vi "set_number_of_channels.vi"(8 "error in (no error)":errorcluster, 10 "number of channels":i32, 11 "GenericImageProcessor.lvclass in":refnum<class "GenericImageProcessor.lvclass">) -> (0 "error out":errorcluster, 3 "GenericImageProcessor.lvclass out":refnum<class "GenericImageProcessor.lvclass">)   [LabVIEW 2010, in "GenericImageProcessor.lvclass"]
uses:
  GenericImageProcessor.lvclass
  GenericImageProcessor.lvclass/GenericImageProcessor.ctl
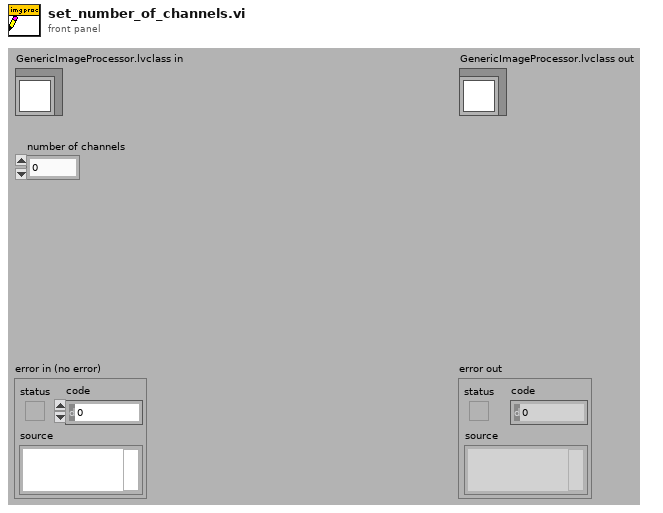
[diagram p1: front panel]
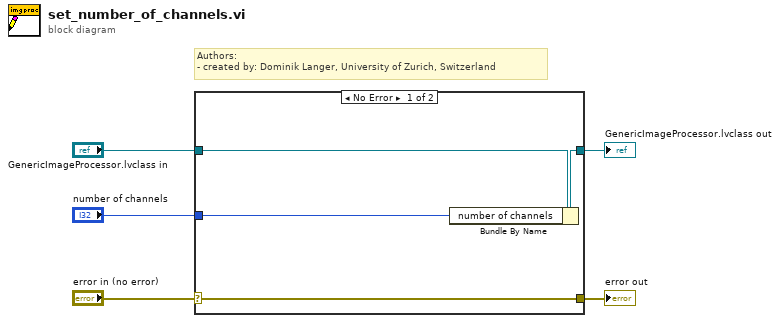
[diagram p0: block diagram]
diagram:
  # "Authors: \n- created by: Dominik Langer, University of Zurich, Switzerland"
  n1 = case shown="No Error" "error in (no error)" {
    selector: "error in (no error)" -> [w9 w10]
    tunnel: [w9 w10] -> w4
    tunnel: [w7 w11] -> w2
    tunnel: "GenericImageProcessor.lvclass in" -> [w8 w11]
    tunnel: "number of channels" -> [w6 _]
    frame No Error {
      n2 = Bundle By Name(cluster=w8, "number of channels"=w6) -> (w7:refnum<class "GenericImageProcessor.lvclass">)
    }
    frame Error {
    }
  }
  "error out" <- w4
  "GenericImageProcessor.lvclass out" <- w2
